vi "高精度时间计数器（秒）.vi"(8 "error in (no error)":errorcluster) -> (0 "error out":errorcluster, 3 "relative seconds":dbl caption="相对秒钟" format="%_19f")   [LabVIEW 2012, in "毫秒定时器.lvlib"]
doc: "Tick Count (ms) primitive with added error handling"
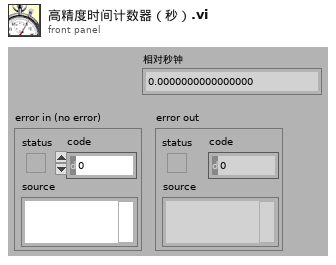
[diagram p1: front panel]
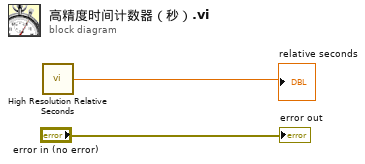
[diagram p0: block diagram]
diagram:
  n1 = call <vilib>:"High Resolution Relative Seconds.vi"() -> ("relative seconds"=→"relative seconds":dbl)
  "error out" <- "error in (no error)"
